vi "lab1 StairClimbing (reference solution).vi"() -> ()   [LabVIEW 2014]
panel:
  out "# of Solutions":i32
  out "Final Solution":i32[][](array[numeric])
  in  "Steps in the stair":i32=5
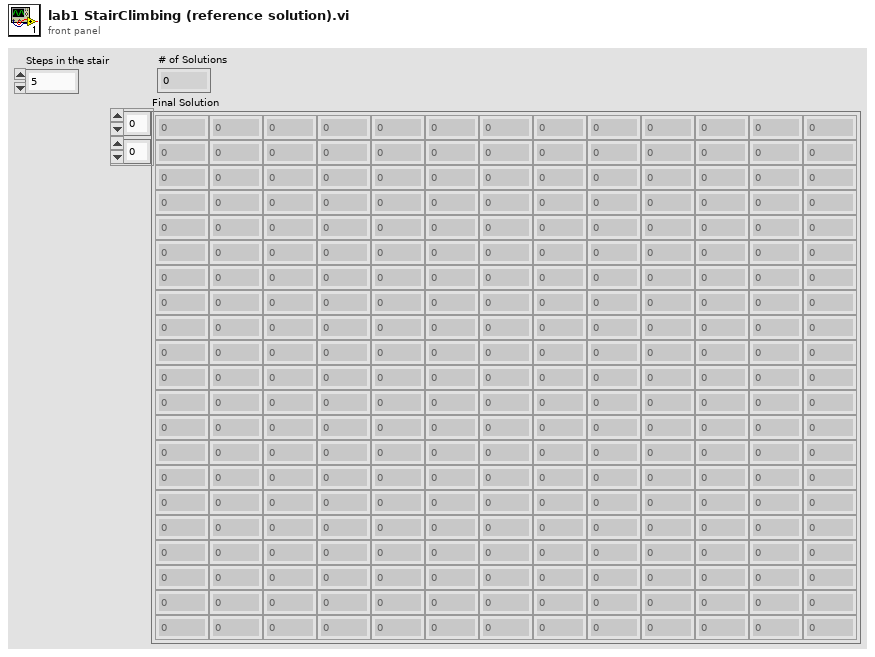
[diagram p1: front panel]
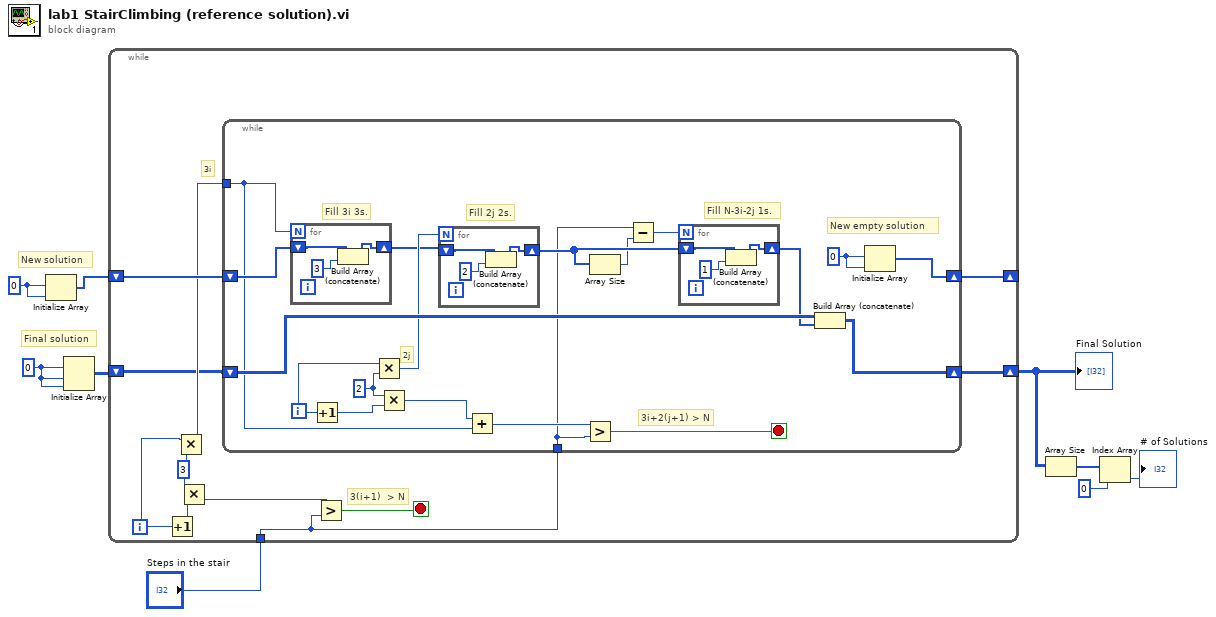
[diagram p0: block diagram]
diagram:
  w6 = 0
  w8 = 0
  # "Final solution"
  # "New solution"
  n1 = Initialize Array(w8, w8) -> (w7:i32[])
  n2 = Initialize Array(w6, w6, w6) -> (w5:i32[][])
  n3 = while {
    tunnel: "Steps in the stair" -> [w14]
    shift-right: [w18] -> w4
    shift-left: w5 -> [w11]
    shift-right: [w19] -> _
    shift-left: w7 -> [w20]
    i -> [w15]
    stop <- w13 stop-if-true
    w10 = 3 ("x")
    # "3i"
    # "3(i+1)  > N"
    n4 = Increment(x=w15) -> (x+1=w17:i32)
    n5 = Multiply(x=w15, y=w10) -> (x*y=w12:i32)
    n6 = Multiply(x=w10, y=w17) -> (x*y=w16:i32)
    n7 = while {
      shift-right: [w24] -> w19
      shift-left: w20 -> [w39]
      shift-right: [w37] -> w18
      shift-left: w11 -> [w38]
      tunnel: w14 -> [w21]
      tunnel: w12 -> [w22]
      i -> [w26]
      stop <- w35 stop-if-true
      w27 = 0
      w25 = 2 ("x")
      # "New empty solution"
      # "Fill N-3i-2j 1s."
      # "Fill 2j 2s."
      # "Fill 3i 3s."
      # "2j"
      # "3i+2(j+1) > N"
      n8 = for {
        N: w22 -> [_]
        shift-right: [w40] -> w28
        shift-left: w39 -> [w42]
        n9 = Build Array (concatenate)(w42, 3) -> (w40:i32[])
      }
      n10 = Increment(x=w26) -> (x+1=w36:i32)
      n11 = Multiply(x=w26, y=w25) -> (x*y=w33:i32)
      n12 = Multiply(x=w25, y=w36) -> (x*y=w23:i32)
      n13 = for {
        N: w33 -> [_]
        shift-right: [w46] -> w32
        shift-left: w28 -> [w48]
        n14 = Build Array (concatenate)(w48, 2) -> (w46:i32[])
      }
      n15 = Add(x=w23, y=w22) -> (x+y=w34:i32)
      n16 = Greater?(x=w34, y=w21) -> (0:w35:bool)
      n17 = Array Size(array=w32) -> (size(s)=w30:i32)
      n18 = Subtract(x=w21, y=w30) -> (x-y=w29:i32)
      n19 = for {
        N: w29 -> [_]
        shift-right: [w43] -> w31
        shift-left: w32 -> [w45]
        n20 = Build Array (concatenate)(w45, 1) -> (w43:i32[])
      }
      n21 = Build Array (concatenate)(w38, w31) -> (w37:i32[][])
      n22 = Initialize Array(w27, w27) -> (w24:i32[])
    }
    n23 = Greater?(x=w16, y=w14) -> (0:w13:bool)
  }
  "Final Solution" <- w4
  n24 = Array Size(array=w4) -> (size(s)=w3:i32[])
  n25 = Index Array(array=w3, index=0) -> (element=→"# of Solutions":i32)
